vi "Cal Progress Bar.vi"() -> ()   [LabVIEW 2016, in "Instrument.Lockin.lvclass"]
uses:
  Instrument.Lockin.lvclass
  <vilib>/addons/WireFlow/_WF_ProgressBar.llb/ProgressBar_WireFlow.lvclass
  <vilib>/addons/WireFlow/_WF_ProgressBar.llb/ProgressBarControlRefs.ctl
panel:
  in  "error in (no error)":errorcluster
  out "error out":errorcluster
  in  "ProgressBar class":refnum<class "ProgressBar_WireFlow.lvclass">
  out "progress":dbl(slide) scale=0.0..100.0
  out "Current message":string="Current item message"
  out "General Message":string="General message"
  in  "Cancel button":bool
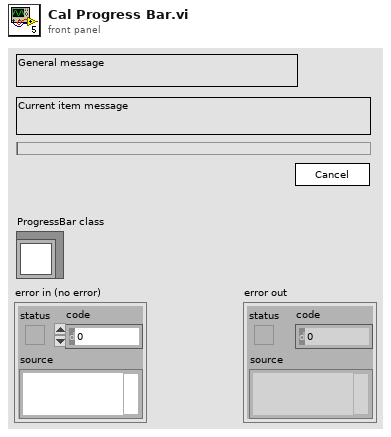
[diagram p1: front panel]
types:
  T1 = typedef "ProgressBar_WireFlow.lvclass/ProgressBarControlRefs.ctl" = cluster{"General message":refnum<vi>, "Current message":refnum<vi>, "Progress value":refnum<vi>, "Cancel Button":refnum<vi>}
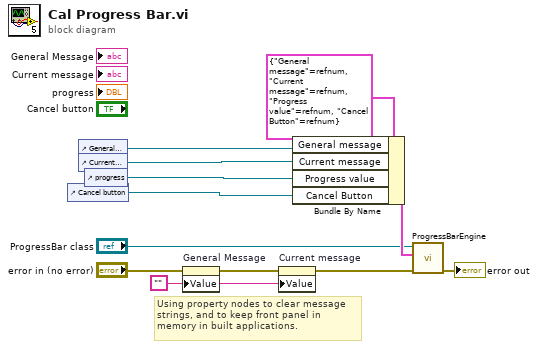
[diagram p0: block diagram]
diagram:
  w11 = ""
  # "Using property nodes to clear message strings, and to keep front panel in memory in built applications."
  n1 = control-ref of="Cancel button"() -> (w12:refnum<vi>)
  n2 = control-ref of="General Message"() -> (w7:refnum<vi>)
  n3 = control-ref of="Current message"() -> (w5:refnum<vi>)
  n4 = control-ref of="progress"() -> (w4:refnum<vi>)
  n5 = property on="General Message" class="Str"(error in="error in (no error)", "Value"=w11) -> (error out=w8:errorcluster)  [unwired: 1 in, 1 out]
  n6 = property on="Current message" class="Str"(error in=w8, "Value"=w11) -> (error out=w10:errorcluster)  [unwired: 1 in, 1 out]
  n7 = Bundle By Name(cluster=T1 {"General message"=refnum, "Current message"=refnum, "Progress value"=refnum, "Cancel Button"=refnum} ("Progress control refs."), "General message"=w7, "Current message"=w5, "Progress value"=w4, "Cancel Button"=w12) -> (w3:T1)
  n8 = call <vilib>:"ProgressBarEngine.vi"("error in (no error)"=w10, "Progress control refs."=w3, "ProgressBar class"="ProgressBar class") -> ("error out"=→"error out":errorcluster)  [unwired: 7 in, 1 out]
